vi "EnableSavePrompt.vi"(3 "Discard shot data":refnum<vi>, 4 "Save shot data":refnum<vi>, 5 "Experiment State in":T1={"error"={"status"=FALSE, "code"=0, "source"=""}, "Digitizer DAQmx Tasks"={"TaskArray"=[]}, "DAQ Settings"={"Channel Settings"=[], "Card Settings"=[]}, "Synchronization Settings"={"Synchronizer 0"="PXI1Slot2", "source terminal"="GlobalSoftwareTrigger", "Synchronizer 1"="PXI1Slot2"}, "DAQ Data"=[], "Next Shot#"="0", "System Message"="", "User Shot Notes"="", "Timing Settings"={"Timing Card Settings"=[], "Timing Channel Settings"=[[{"Delay (s)"=2.559999942779541, "Pulse width (s)"=0.009999999776482582, "Active"=TRUE, "Channel Name"="Fiber 8", "counter"="PXI1Slot8/ctr7", "FrontPanelTime"=2.559999942779541}]]}, "Timing Tasks"={"TaskArray"=[]}, "Tree"="0", "Time Card/Channels"=[2, 8], "DAQ Card/Channels"=[3, 8], "Program Version"="", "RIO Settings"={"Channel Settings"=[], "Card Settings"=[]}, "RIO References"={"Reference Array"=[]}, "RIO Data"={"RIO Deleaved Data"=[], "Raw Readout"=[]}, "RIO Card/Channels"=[3, 8], "DIO Channels"=0, "DIO Settings"={"DIO Channel Array"=[]}, "Tachometer Controls"={"Tach Calibration folder"=path "Z:/Data/Calibration/Tachometer", "PSU2 charging Voltage [kV]"=0.0, "PSU2 Counter"="", "PSU3 Counter"="", "PSU3 charging Voltage [kV]"=0.0}, "Global Settings"={"Initial Background Values"={"Reference Shot #"=0.0, "Background pressure [Torr]"=0.0, "Cryo temp [V]"=0.0, "Cryo temp [K]"=0.0, "Cryotemp Calibration File"=path ""}, "Gas Puffing"={"Gas A type"="N", "Gas B type"="N", "Gas C type"="N", "Gas A pressure [psi]"=0.0, "Gas B pressure [psi]"=0.0, "Gas C pressure [psi]"=0.0, "Innner Electrode"="", "Middle Electrode"="", "Outer Electrode"="", "Gas A bottle pressure [psi]"=0.0, "Gas B bottle pressure [psi]"=0.0, "Gas C bottle pressure [psi]"=0.0}, "PSU Voltages"={"Bias1 Voltage [V]"=0.0, "Bias2 Voltage [V]"=0.0, "PSU1 Voltage [V]"=0.0, "Puff-PSU1 CH1 Voltage [V]"=0.0, "Puff-PSU1 CH2 Voltage [V]"=0.0, "Puff-PSU1 CH3 Voltage [V]"=0.0}, "Scope Details"={"CH1"="", "CH2"="", "CH3"="", "CH4"="", "CH1 Ground State"="Grounded", "CH2 Ground State"="Grounded", "CH3 Ground State"="Grounded", "CH4 Ground State"="Grounded"}}, "Calibrations"={"CryoTemp"={"Comment"="", "X"=[], "Y"=[]}, "PSU2 Tach"={"Comment"="", "X"=[], "Y"=[]}, "PSU3 Tach"={"Comment"="", "X"=[], "Y"=[]}}, "Tach Tasks"={"PSU2 task"="", "PSU3 task"=""}} {"Global Settings"."Initial Background Values"."Cryo temp [K]" format="%#_4g"; "RIO Settings"."Card Settings"."Sample Rate" format="%#_3p"; "Timing Settings"."Timing Channel Settings"."FrontPanelTime" format="%.3p"; "Timing Settings"."Timing Channel Settings"."Pulse width (s)" format="%.3p"; "Timing Settings"."Timing Channel Settings"."Delay (s)" format="%.3p"; "DAQ Settings"."Card Settings"."Global Edge Type" items=["Rising"=10280, "Falling"=10171]; "DAQ Settings"."Card Settings"."Sample Rate" format="%#_3p"}) -> (2 "Experiment State out":T1={"error"={"status"=FALSE, "code"=0, "source"=""}, "Digitizer DAQmx Tasks"={"TaskArray"=[]}, "DAQ Settings"={"Channel Settings"=[], "Card Settings"=[]}, "Synchronization Settings"={"Synchronizer 0"="PXI1Slot2", "source terminal"="GlobalSoftwareTrigger", "Synchronizer 1"="PXI1Slot2"}, "DAQ Data"=[], "Next Shot#"="0", "System Message"="", "User Shot Notes"="", "Timing Settings"={"Timing Card Settings"=[], "Timing Channel Settings"=[[{"Delay (s)"=2.559999942779541, "Pulse width (s)"=0.009999999776482582, "Active"=TRUE, "Channel Name"="Fiber 8", "counter"="PXI1Slot8/ctr7", "FrontPanelTime"=2.559999942779541}]]}, "Timing Tasks"={"TaskArray"=[]}, "Tree"="0", "Time Card/Channels"=[2, 8], "DAQ Card/Channels"=[3, 8], "Program Version"="", "RIO Settings"={"Channel Settings"=[], "Card Settings"=[]}, "RIO References"={"Reference Array"=[]}, "RIO Data"={"RIO Deleaved Data"=[], "Raw Readout"=[]}, "RIO Card/Channels"=[3, 8], "DIO Channels"=0, "DIO Settings"={"DIO Channel Array"=[]}, "Tachometer Controls"={"Tach Calibration folder"=path "Z:/Data/Calibration/Tachometer", "PSU2 charging Voltage [kV]"=0.0, "PSU2 Counter"="", "PSU3 Counter"="", "PSU3 charging Voltage [kV]"=0.0}, "Global Settings"={"Initial Background Values"={"Reference Shot #"=0.0, "Background pressure [Torr]"=0.0, "Cryo temp [V]"=0.0, "Cryo temp [K]"=0.0, "Cryotemp Calibration File"=path ""}, "Gas Puffing"={"Gas A type"="N", "Gas B type"="N", "Gas C type"="N", "Gas A pressure [psi]"=0.0, "Gas B pressure [psi]"=0.0, "Gas C pressure [psi]"=0.0, "Innner Electrode"="", "Middle Electrode"="", "Outer Electrode"="", "Gas A bottle pressure [psi]"=0.0, "Gas B bottle pressure [psi]"=0.0, "Gas C bottle pressure [psi]"=0.0}, "PSU Voltages"={"Bias1 Voltage [V]"=0.0, "Bias2 Voltage [V]"=0.0, "PSU1 Voltage [V]"=0.0, "Puff-PSU1 CH1 Voltage [V]"=0.0, "Puff-PSU1 CH2 Voltage [V]"=0.0, "Puff-PSU1 CH3 Voltage [V]"=0.0}, "Scope Details"={"CH1"="", "CH2"="", "CH3"="", "CH4"="", "CH1 Ground State"="Grounded", "CH2 Ground State"="Grounded", "CH3 Ground State"="Grounded", "CH4 Ground State"="Grounded"}}, "Calibrations"={"CryoTemp"={"Comment"="", "X"=[], "Y"=[]}, "PSU2 Tach"={"Comment"="", "X"=[], "Y"=[]}, "PSU3 Tach"={"Comment"="", "X"=[], "Y"=[]}}, "Tach Tasks"={"PSU2 task"="", "PSU3 task"=""}} {"Global Settings"."Initial Background Values"."Cryo temp [K]" format="%#_4g"; "RIO Settings"."Card Settings"."Sample Rate" format="%#_3p"; "Timing Settings"."Timing Channel Settings"."FrontPanelTime" format="%.3p"; "Timing Settings"."Timing Channel Settings"."Pulse width (s)" format="%.3p"; "Timing Settings"."Timing Channel Settings"."Delay (s)" format="%.3p"; "DAQ Settings"."Card Settings"."Global Edge Type" items=["Rising"=10280, "Falling"=10171]; "DAQ Settings"."Card Settings"."Sample Rate" format="%#_3p"})   [LabVIEW 2014]
doc: "Enable Save and discard buttons in order to allow user to specify wether or not the shot is to be saved."
uses:
  Controls/ExperimentStateCluster.ctl
  Controls/DigitizerSettingsChannelSettings.ctl
  Controls/DigitizerSettingsCardSettingsArray.ctl
  Controls/DigitizerSettingsCardSettings.ctl
  Controls/TimingSettings.ctl
  Controls/TimingCardSettings.ctl
  Controls/TimingChannelSettings.ctl
  Controls/RIOSettingsExperimentStateCluster.ctl
  Controls/RIOChannelSettingsArrayExperimentStateCluster.ctl
  Controls/RIOSettingsChannelSettings.ctl
  Controls/RIOSettingsCardSettingsArray.ctl
  Controls/RIOSettingsCardSettings.ctl
  <vilib>/userdefined/High Color/nirio_resource_hc.ctl
  Controls/RIOData.ctl
  Controls/DIOChannel.ctl
  Controls/TachometerControls.ctl
  Controls/Global Settings/GlobalSettings.ctl
  Controls/Global Settings/InitialBackgroundValues.ctl
  Controls/Global Settings/GasPuffing.ctl
  Controls/Global Settings/PSUVoltages.ctl
  Controls/Global Settings/ScopeDetails.ctl
  Controls/Calibrations/Calibrations.ctl
  Controls/Calibrations/CryoTemoCalibration.ctl
  Controls/Calibrations/PSU2TachCalibration.ctl
  Controls/Calibrations/PSU3TachCalibration.ctl
  Controls/TachTasks.ctl
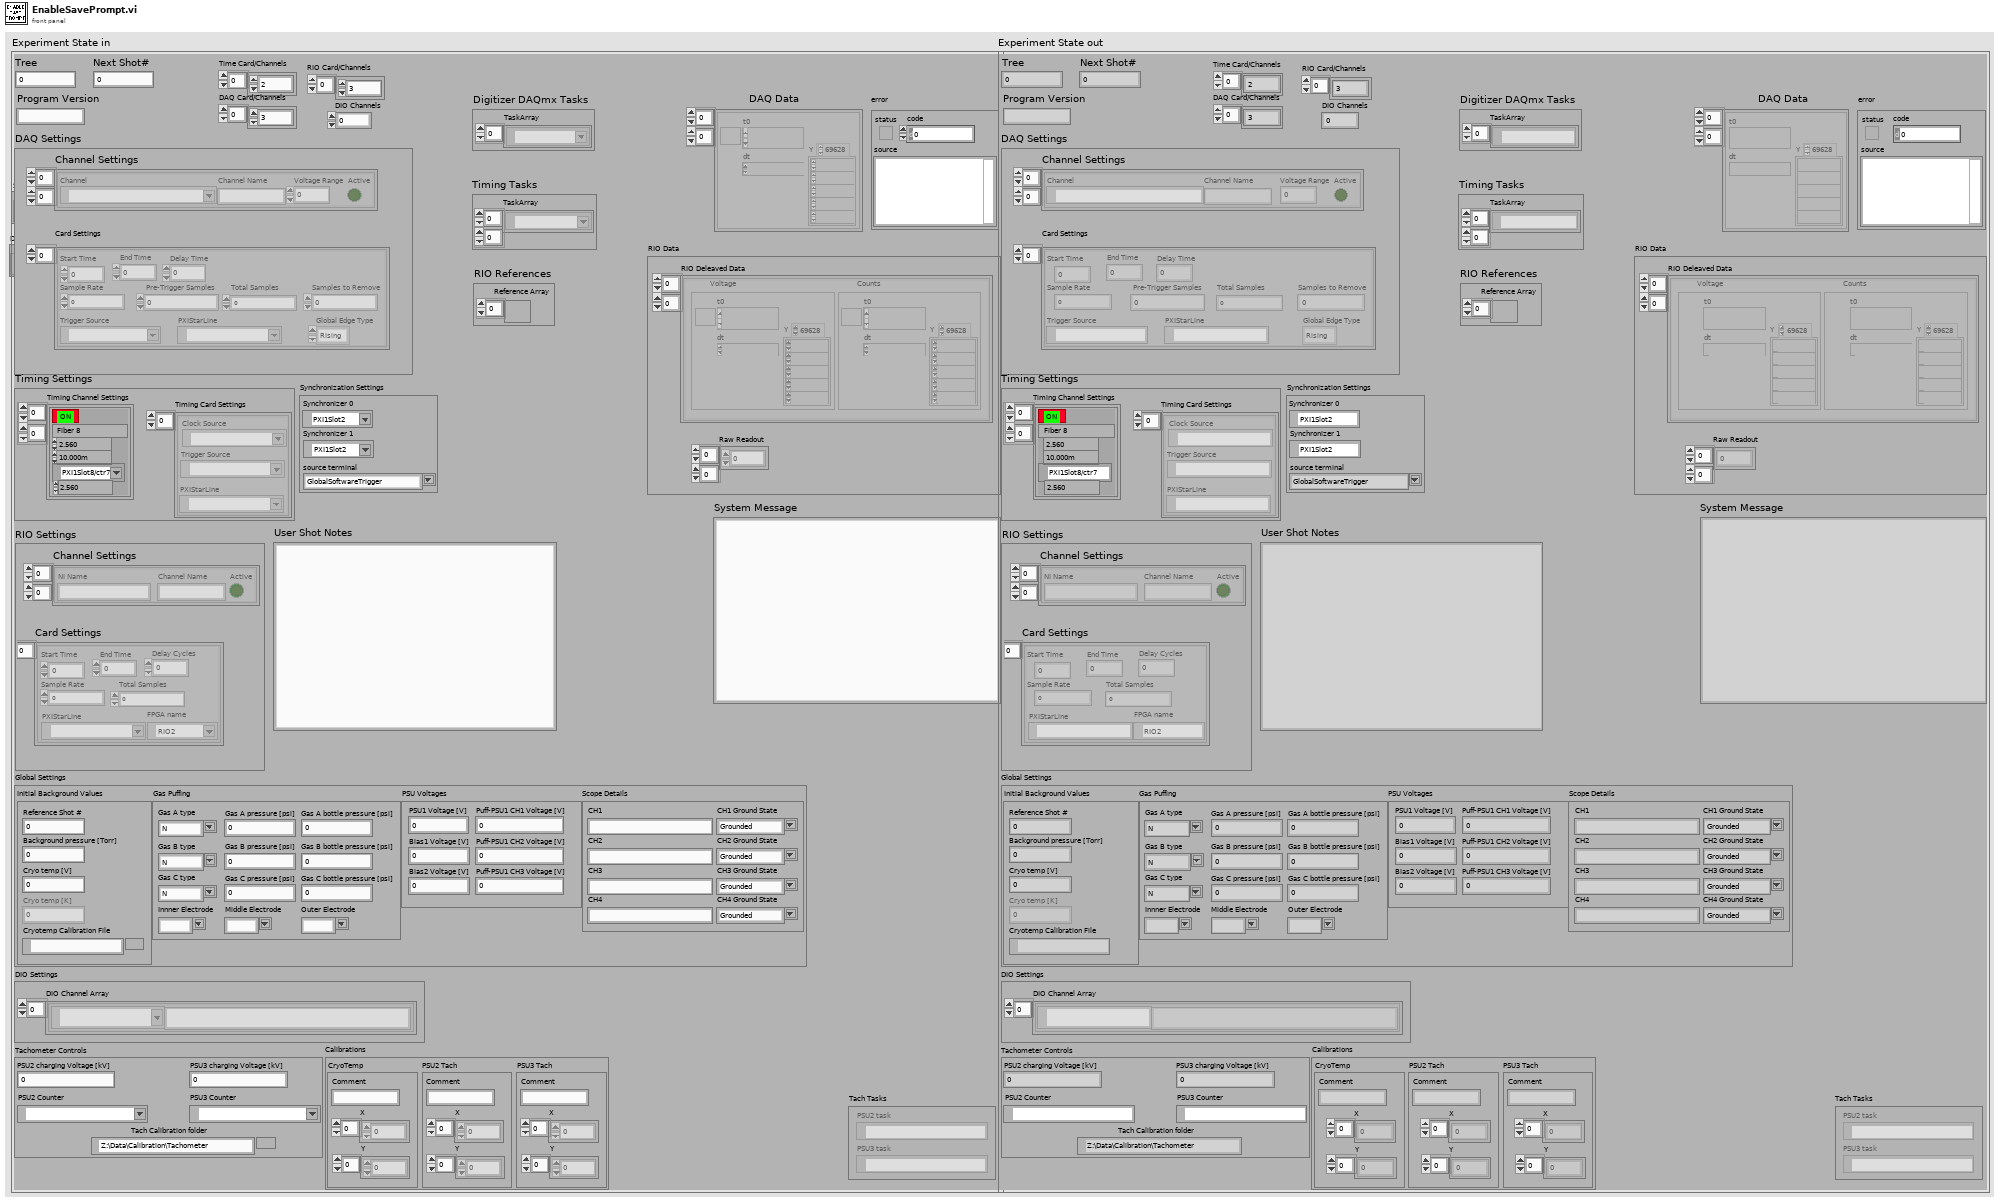
[diagram p1: front panel]
types:
  T1 = typedef "ExperimentStateCluster.ctl" = cluster{"error":errorcluster, "Digitizer DAQmx Tasks":cluster{"TaskArray":refnum<k21>[]}, "DAQ Settings":cluster{"Channel Settings":T2[][], "Card Settings":T3}, "Synchronization Settings":cluster{"Synchronizer 0":refnum<k15>, "source terminal":string, "Synchronizer 1":refnum<k15>}, "DAQ Data":waveform(dbl)[][], "Next Shot#":string, "System Message":string, "User Shot Notes":string, "Timing Settings":T5, "Timing Tasks":cluster{"TaskArray":refnum<k21>[][]}, "Tree":string, "Time Card/Channels":i32[], "DAQ Card/Channels":i32[], "Program Version":string, "RIO Settings":T8, "RIO References":cluster{"Reference Array":refnum<k20>[]}, "RIO Data":T14, "RIO Card/Channels":i32[], "DIO Channels":i32, "DIO Settings":cluster{"DIO Channel Array":T15[]}, "Tachometer Controls":T16, "Global Settings":T17, "Calibrations":T22, "Tach Tasks":T26}
  T2 = typedef "DigitizerSettingsChannelSettings.ctl" = cluster{"Channel":tag, "Channel Name":string, "Voltage Range":dbl, "Active":bool}
  T3 = typedef "DigitizerSettingsCardSettingsArray.ctl" = T4[]
  T4 = typedef "DigitizerSettingsCardSettings.ctl" = cluster{"Start Time":dbl, "End Time":dbl, "Sample Rate":dbl, " Pre-Trigger Samples":u32, "Total Samples":i32, "Samples to Remove":u32, "Trigger Source":tag, "Global Edge Type":i32, "PXIStarLine":tag, "Delay Time":dbl}
  T5 = typedef "TimingSettings.ctl" = cluster{"Timing Card Settings":T6[], "Timing Channel Settings":T7[][]}
  T6 = typedef "TimingCardSettings.ctl" = cluster{"Trigger Source":tag, "Clock Source":tag, "PXIStarLine":tag}
  T7 = typedef "TimingChannelSettings.ctl" = cluster{"Delay (s)":dbl, "Pulse width (s)":dbl, "Active":bool, "Channel Name":string, "counter":tag, "FrontPanelTime":dbl}
  T8 = typedef "RIOSettingsExperimentStateCluster.ctl" = cluster{"Channel Settings":T9, "Card Settings":T11}
  T9 = typedef "RIOChannelSettingsArrayExperimentStateCluster.ctl" = T10[][]
  T10 = typedef "RIOSettingsChannelSettings.ctl" = cluster{"Channel Name":string, "Active":bool, "NI Name":string}
  T11 = typedef "RIOSettingsCardSettingsArray.ctl" = T12[]
  T12 = typedef "RIOSettingsCardSettings.ctl" = cluster{"Start Time":dbl, "End Time":dbl, "Sample Rate":dbl, "Total Samples":u64, "PXIStarLine":tag, "Delay Cycles":u64, "FPGA name":T13}
  T13 = typedef "nirio_resource_hc.ctl" = tag
  T14 = typedef "RIOData.ctl" = cluster{"RIO Deleaved Data":cluster{"Voltage":waveform(dbl), "Counts":waveform(i16)}[][], "Raw Readout":u64[][]}
  T15 = typedef "DIOChannel.ctl" = cluster{"Channel Name":string, "NI Name":tag}
  T16 = typedef "TachometerControls.ctl" = cluster{"Tach Calibration folder":path, "PSU2 charging Voltage [kV]":dbl, "PSU2 Counter":tag, "PSU3 Counter":tag, "PSU3 charging Voltage [kV]":dbl}
  T17 = typedef "GlobalSettings.ctl" = cluster{"Initial Background Values":T18, "Gas Puffing":T19, "PSU Voltages":T20, "Scope Details":T21}
  T18 = typedef "InitialBackgroundValues.ctl" = cluster{"Reference Shot #":dbl, "Background pressure [Torr]":dbl, "Cryo temp [V]":dbl, "Cryo temp [K]":dbl, "Cryotemp Calibration File":path}
  T19 = typedef "GasPuffing.ctl" = cluster{"Gas A type":string, "Gas B type":string, "Gas C type":string, "Gas A pressure [psi]":dbl, "Gas B pressure [psi]":dbl, "Gas C pressure [psi]":dbl, "Innner Electrode":string, "Middle Electrode":string, "Outer Electrode":string, "Gas A bottle pressure [psi]":dbl, "Gas B bottle pressure [psi]":dbl, "Gas C bottle pressure [psi]":dbl}
  T20 = typedef "PSUVoltages.ctl" = cluster{"Bias1 Voltage [V]":dbl, "Bias2 Voltage [V]":dbl, "PSU1 Voltage [V]":dbl, "Puff-PSU1 CH1 Voltage [V]":dbl, "Puff-PSU1 CH2 Voltage [V]":dbl, "Puff-PSU1 CH3 Voltage [V]":dbl}
  T21 = typedef "ScopeDetails.ctl" = cluster{"CH1":string, "CH2":string, "CH3":string, "CH4":string, "CH1 Ground State":string, "CH2 Ground State":string, "CH3 Ground State":string, "CH4 Ground State":string}
  T22 = typedef "Calibrations.ctl" = cluster{"CryoTemp":T23, "PSU2 Tach":T24, "PSU3 Tach":T25}
  T23 = typedef "CryoTemoCalibration.ctl" = cluster{"Comment":string, "X":dbl[], "Y":dbl[]}
  T24 = typedef "PSU2TachCalibration.ctl" = cluster{"Comment":string, "X":dbl[], "Y":dbl[]}
  T25 = typedef "PSU3TachCalibration.ctl" = cluster{"Comment":string, "X":dbl[], "Y":dbl[]}
  T26 = typedef "TachTasks.ctl" = cluster{"PSU2 task":refnum<k21>, "PSU3 task":refnum<k21>}
  T27 = enum8{"Enabled", "Disabled", "Disabled and Grayed Out"}
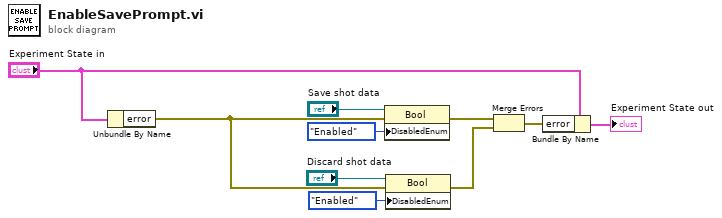
[diagram p0: block diagram]
diagram:
  n1 = Unbundle By Name("Experiment State in") -> ("error"=w2:errorcluster)
  n2 = property class="Bool"(reference="Save shot data", error in=w2, "DisabledEnum"=T27."Enabled" ("Disabled")) -> (error out=w4:errorcluster)  [unwired: 1 out]
  n3 = property class="Bool"(reference="Discard shot data", error in=w2, "DisabledEnum"=T27."Enabled" ("Disabled")) -> (error out=w3:errorcluster)  [unwired: 1 out]
  n4 = Merge Errors(w4, w3) -> (w5:errorcluster)
  n5 = Bundle By Name(cluster="Experiment State in", "error"=w5) -> (→"Experiment State out":T1)
